vi "Scanner with R and T displays.vi"() -> ()   [LabVIEW 2012]
doc: "Application example"
uses:
  <vilib>/ptbypt/NI_PtbyPt.lvlib
panel:
  in  "EXIT W/O SAVING":bool
  out "MEASURING":i32
  out "EDIT":string
  out "SELECT":string
  out "SCAN CYCLE FINISHED":bool
  out "ADC OVERRANGE":bool
  out "UNIT":string[](array[string])
  out "RPC7":bool
  out "RPC6":bool
  out "RPC5":bool
  out "RPC4":bool
  out "RPC3":bool
  out "RPC2":bool
  out "RPC1":bool
  out "RPC0":bool
  out "T[CH]":dbl[](array[numeric]) format="%_6g"
  out "RPC":bool[](array[boolean])
  out "CURRENT TEMPERATURE":dbl caption="TEMPERATURE" format="%_5f"
  out "CH0":bool
  out "CH1":bool
  out "CH2":bool
  out "CH3":bool
  out "CH4":bool
  out "CH5":bool
  out "CH6":bool
  out "CH7":bool
  out "R[CH] OHMS":dbl[](array[numeric]) format="%_6g"
  in  "RESISTANCE":dbl format="%_5f"
  in  "SCAN SETTINGS":T1(array[cluster])=[{"SCAN ENABLED"=0, "INPUT"=0, "RANGE"=3, "AUTORANGE"=0, "EXCITATION"=0, "STAB DELAY"=0, "AVERAGE COUNT"=1}, {"SCAN ENABLED"=0, "INPUT"=0, "RANGE"=3, "AUTORANGE"=0, "EXCITATION"=0, "STAB DELAY"=0, "AVERAGE COUNT"=1}, {"SCAN ENABLED"=0, "INPUT"=0, "RANGE"=3, "AUTORANGE"=0, "EXCITATION"=0, "STAB DELAY"=0, "AVERAGE COUNT"=1}, {"SCAN ENABLED"=0, "INPUT"=0, "RANGE"=3, "AUTORANGE"=0, "EXCITATION"=0, "STAB DELAY"=0, "AVERAGE COUNT"=1}, {"SCAN ENABLED"=0, "INPUT"=0, "RANGE"=3, "AUTORANGE"=0, "EXCITATION"=0, "STAB DELAY"=0, "AVERAGE COUNT"=1}, {"SCAN ENABLED"=0, "INPUT"=0, "RANGE"=3, "AUTORANGE"=0, "EXCITATION"=0, "STAB DELAY"=0, "AVERAGE COUNT"=1}, {"SCAN ENABLED"=0, "INPUT"=0, "RANGE"=3, "AUTORANGE"=0, "EXCITATION"=0, "STAB DELAY"=0, "AVERAGE COUNT"=1}, {"SCAN ENABLED"=0, "INPUT"=0, "RANGE"=3, "AUTORANGE"=0, "EXCITATION"=0, "STAB DELAY"=0, "AVERAGE COUNT"=1}] {"SCAN ENABLED" items=["NO", "YES"]; "INPUT" items=["ZERO", "MEAS", "CAL"]; "RANGE" items=["NO RANGE", "2 Ohms", "20 Ohms", "200 Ohms", "2 kOhms", "20 kOhms", "200 kOhms", "2 MOhms"]; "AUTORANGE" items=["NO", "YES"]; "EXCITATION" items=["NO EXCITATION", "3 uV", "10uV", "30uV", "100uV", "300uV", "1mV", "3mV"]}
  in  "STOP":bool caption="PREMATURE STOPPING"
  in  "CH":i32
  in  "AVG_I":i32
  in  "START A CYCLE":bool
  in  "EXIT AND SAVE":bool
  out "SCAN FILE READ INFO":string
  # "Scanner with R and T Displays.vi"
  # "CURRENTLY MEASURING"
  # "CH"
  # "Start the VI before editing. Edits\nmade before starting are lost."
  # "R Past Calibration\nRange"
  # "Prepare the R/T calibration text files according to instructions\nPrepare information file about the calibration files using Edit RT Information File.vi\nTest the R/T conversion using Free Running Avs47b with temperature display.vi \n\nStart this VI. SCAN FILE READ INFO will be blank, if all the calibration files that are\nlisted by file avs47b_rt_file_info.cnf . \"Select Action..\" -text  should appear.\nEdit the scan settings, if needed. Enable scanning for the required channels, select suitable  \nrange and excitation for those channels. \n\n If possible, enable autoranging for each channel that will be scanned. This will prevent \nresults that include erroneous readings due to ADC overload.  After starting, autoranging\ncontinues until a valid range is found.  Then the channel is measured. If the reading\nfalls under 1800 or exceeds 19000 during averaging, range is changed downwards or\nupwards and, after a stabilisation delay, averaging starts from the beginning.\n\nStabilisation delay should be about 5 seconds for the highest excitations and about 15 \nseconds for the lowest excitation. There is a tradeoff between scanning speed and \ntime for finding good and final balance.  Required average count depends on excitation \nand the desired accuracy. \n\nWhen you are ready with editing, either save the edited (or non-edited) settings and exit, \nor start a single scan cycle. The settings will be saved after the cycle.\n\nThe scan-enabled channels are measured.  The mean values of resistances\nare output for all channels, temperatures are shown for channels that have a \ncalibration file.  Temperature unit has been specified in the scan info file.\nAfter the scan cycle, the bridge returns to its initial state. The possibly edited\nscan settings are saved."
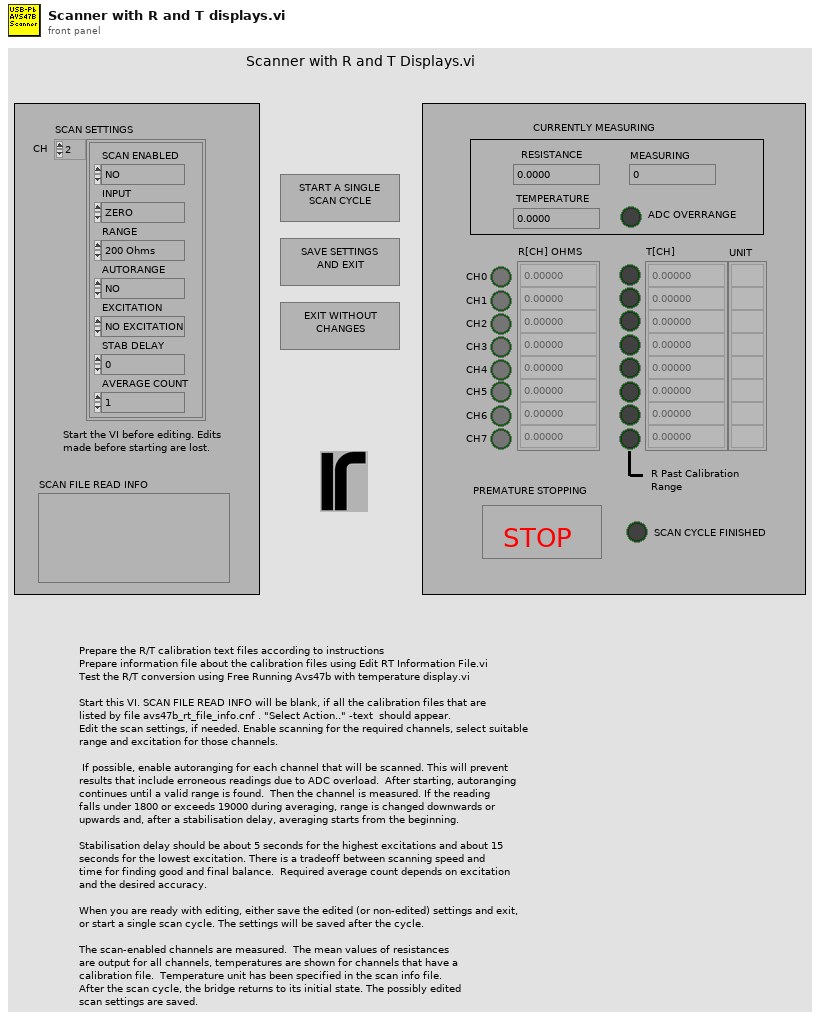
[diagram p1: front panel]
types:
  T1 = cluster{"SCAN ENABLED":u8, "INPUT":u8, "RANGE":u8, "AUTORANGE":u8, "EXCITATION":u8, "STAB DELAY":i32, "AVERAGE COUNT":i32}[]
  T2 = enum16{"NONE", "READ", "READ AND EDIT", "DEFAULTS"}
  T3 = cluster{"VISA RESOURCE":refnum<visa-resource-name>, "PICOBUS ADDRESS":u8, "DISABLE AL":u8, "REMOTE":u8, "INPUT":u8, "CHANNEL":u8, "RANGE":u8, "EXCITATION":u8, "DISPLAY":u8, "DIGITAL REFERENCE":u16, "SET POINT":dbl, "PROP GAIN":u8, "INTG":u8, "DERIV":u8, "POWER BIAS":u8, "POWER RANGE":u8, "INFO STRING":string, "HEATER RESISTANCE":dbl, "INTERVAL":u8, " SENSOR dR/dT":u8}
  T4 = cluster{"NUMBER OF POINTS":i32, "SIGN OF dT/dR":enum16{"POSITIVE", "NEGATIVE"}, "R/T FORMAT ":enum16{"R", "LOG(R)"}, "TEMPERATURE SCALE":enum16{"KELVINS", "CELSIUS"}, "FILE OK":i32}[]
  T5 = enum16{"SCAN CHECK", "CONFIGURE", "MEASURE", "CALC AVE", "READY"}
  T6 = cluster{"SCAN ENABLED":u8, "INPUT":u8, "RANGE":u8, "AUTORANGE":u8, "EXCITATION":u8, "STAB DELAY":i32, "AVERAGE COUNT":i32}
  T7 = cluster{bool, bool, bool, bool, bool, bool, bool, bool, bool, bool, bool, bool, bool, bool, bool, bool}
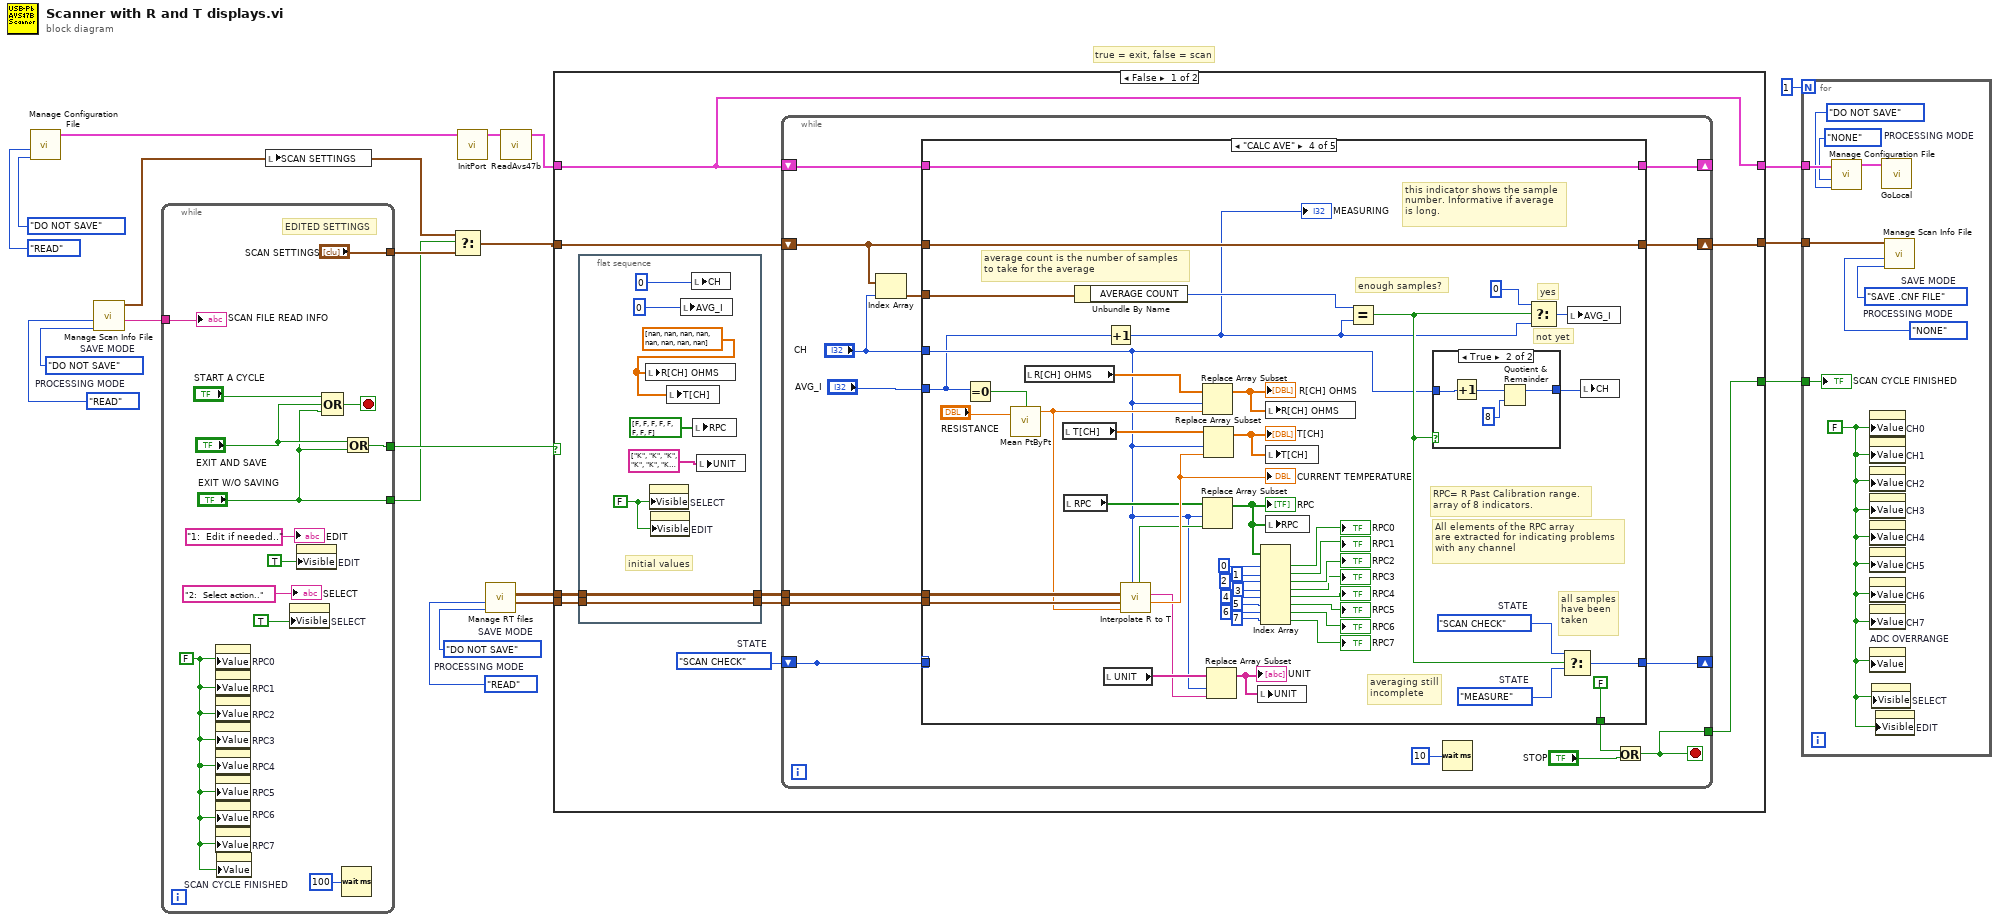
[diagram p0: block diagram]
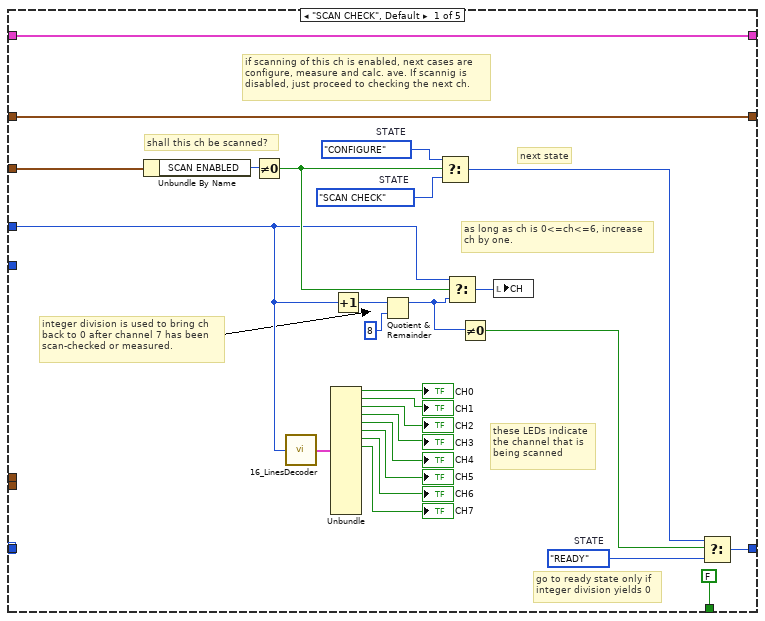
[diagram p2: hidden frame]
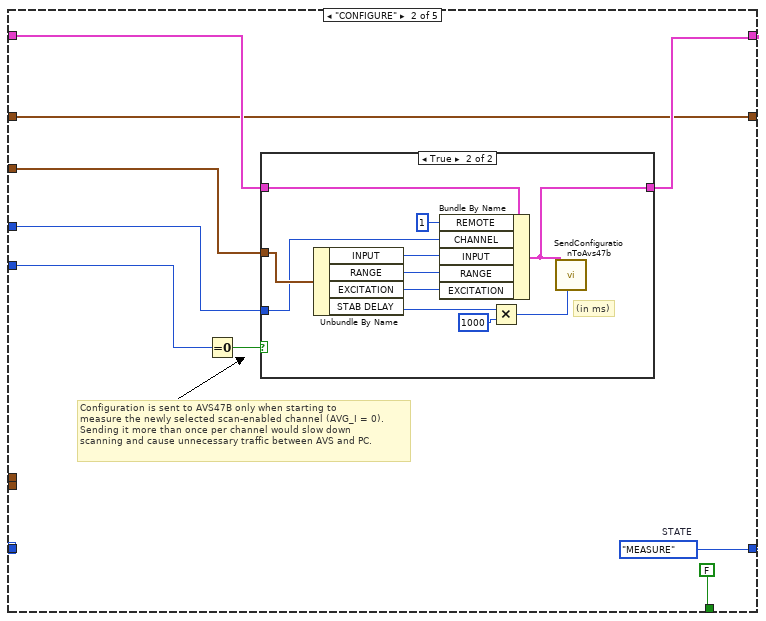
[diagram p3: hidden frame]
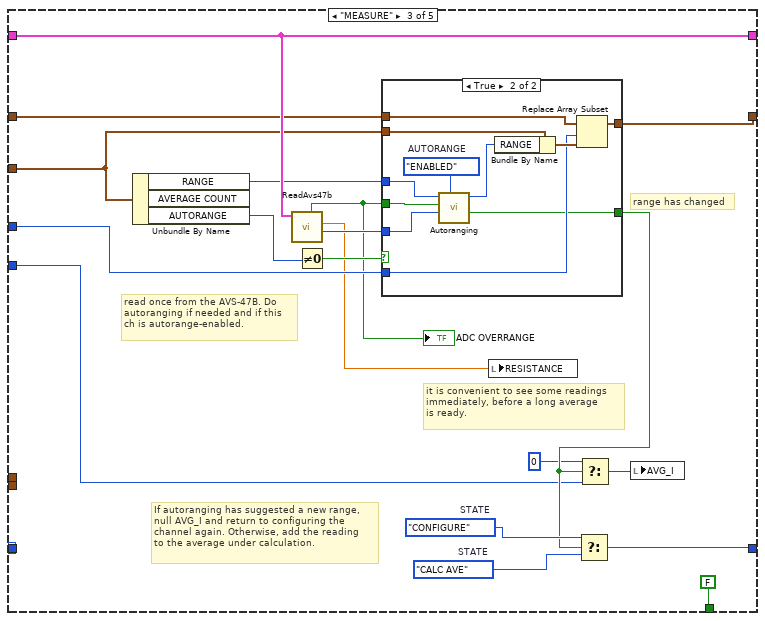
[diagram p5: hidden frame]
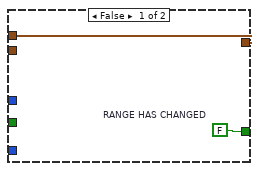
[diagram p6: hidden frame]
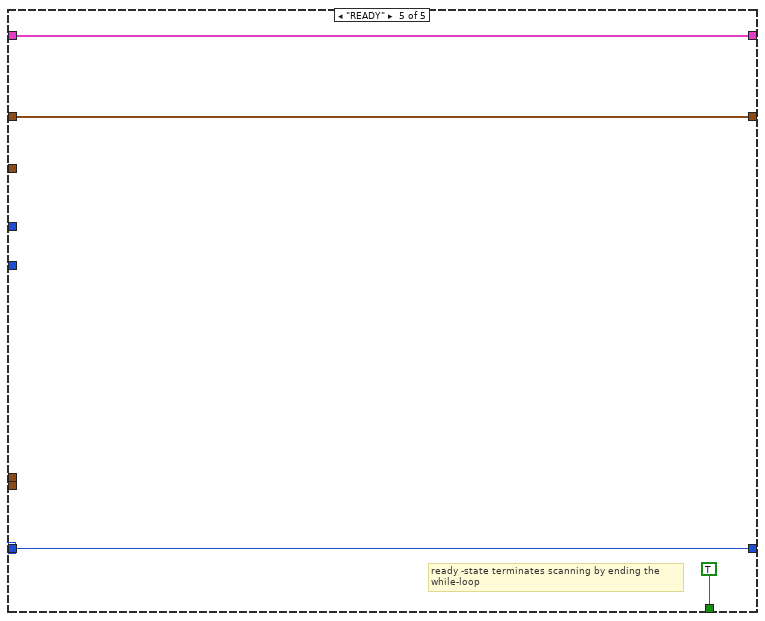
[diagram p8: hidden frame]
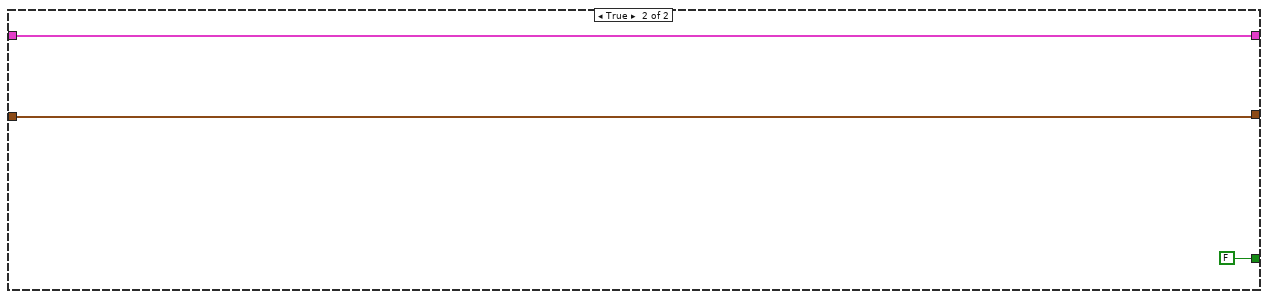
[diagram p9: hidden frame]
diagram:
  w6 = T2."READ"  # PROCESSING MODE
  w7 = enum16{"DO NOT SAVE", "SAVE .CNF FILE"}."DO NOT SAVE"  # SAVE MODE
  w10 = T2."READ"  # PROCESSING MODE
  w11 = enum16{"DO NOT SAVE", "SAVE .CNF FILE"}."DO NOT SAVE"  # SAVE MODE
  # "true = exit, false = scan"
  n1 = call "Manage Configuration File.vi"("SAVE MODE"=enum16{"DO NOT SAVE", "SAVE .CNF FILE"}."DO NOT SAVE", "PROCESSING MODE"=enum16{"NONE", "READ", "CREATE"}."READ") -> ("CONFIGURATION CLUSTER OUT"=w5:T3)  [unwired: 9 in]
  n2 = call "Manage Scan Info File.vi"("SAVE MODE"=w11, "PROCESSING MODE"=w10) -> ("SCAN FILE READ INFO"=w12:string, "SCAN INFO CLUSTER ARRAY OUT"=w3:T1)  [unwired: 7 in, 1 out]
  n3 = while {
    tunnel: [w24] -> w21
    tunnel: ["SCAN SETTINGS"] -> w4
    tunnel: w12 -> [w33]
    tunnel: ["EXIT W/O SAVING"] -> w2
    stop <- w26 stop-if-true
    w27 = FALSE ("RPC0")
    # "EDITED SETTINGS"
    n4 = property on="RPC0" class="Bool (strict)"("Value"=w27) -> ()  [unwired: 2 in, 2 out]
    n5 = property on="RPC1" class="Bool (strict)"("Value"=w27) -> ()  [unwired: 2 in, 2 out]
    n6 = property on="RPC2" class="Bool (strict)"("Value"=w27) -> ()  [unwired: 2 in, 2 out]
    n7 = property on="RPC3" class="Bool (strict)"("Value"=w27) -> ()  [unwired: 2 in, 2 out]
    n8 = property on="RPC4" class="Bool (strict)"("Value"=w27) -> ()  [unwired: 2 in, 2 out]
    n9 = property on="RPC5" class="Bool (strict)"("Value"=w27) -> ()  [unwired: 2 in, 2 out]
    n10 = property on="RPC6" class="Bool (strict)"("Value"=w27) -> ()  [unwired: 2 in, 2 out]
    n11 = property on="RPC7" class="Bool (strict)"("Value"=w27) -> ()  [unwired: 2 in, 2 out]
    n12 = property on="SCAN CYCLE FINISHED" class="Bool (strict)"("Value"=w27) -> ()  [unwired: 2 in, 2 out]
    n13 = property on="SELECT" class="Str"("Visible"=TRUE) -> ()  [unwired: 2 in, 2 out]
    n14 = property on="EDIT" class="Str"("Visible"=TRUE) -> ()  [unwired: 2 in, 2 out]
    n15 = Compound Arithmetic op=OR("START A CYCLE", "EXIT AND SAVE", "EXIT W/O SAVING") -> (w26:bool)
    n16 = Wait (ms)(milliseconds to wait=u32 100) -> ()  [unwired: 1 out]
    n17 = Or(x="EXIT AND SAVE", y="EXIT W/O SAVING") -> (x .or. y?=w24:bool)
    "SCAN FILE READ INFO" <- w33
    "EDIT" <- "1:  Edit if needed.."
    "SELECT" <- "2:  Select action.."
  }
  n18 = local write "SCAN SETTINGS"(w3) -> ()
  n19 = Select(t=w3, s=w2, f=w4) -> (s? t:f=w1:T1)
  n20 = call "InitPort.vi"("CONFIGURATION CLUSTER"=w5) -> ("UNMODIFIED CONFIGURATION CLUSTER"=w13:T3)  [unwired: 6 in, 2 out]
  n21 = call "Manage RT files.vi"("SAVE MODE"=w7, "PROCESSING MODE"=w6) -> ("FILE INFO"=w8:T4, "R/T BREAKPOINTS"=w9:cluster{dbl, dbl}[][])  [unwired: 5 in, 3 out]
  n22 = call "ReadAvs47b.vi"("CONFIGURATION CLUSTER"=w13) -> ("MODIFIED CONFIGURATION CLUSTER"=w16:T3)  [unwired: 5 in, 5 out]
  n23 = case shown="False" w21 {
    tunnel: w1 -> [w36 w203]
    tunnel: w16 -> [w42 w204]
    tunnel: [w42 w204] -> w20
    tunnel: [w35 w203] -> w19
    tunnel: w9 -> [w41 _]
    tunnel: w8 -> [w39 _]
    tunnel: [w37 FALSE] -> w17
    frame False {
      w43 = T5."SCAN CHECK"  # STATE
      n24 = flat-sequence {
        tunnel: w41 -> [w47]
        tunnel: [w47] -> w40
        tunnel: w39 -> [w46]
        tunnel: [w46] -> w38
        frame #0 {
          w44 = FALSE ("Visible")
          w49 = dbl[] [nan, nan, nan, nan, nan, nan, nan, nan]
          # "initial values"
          n25 = local write "R[CH] OHMS"(w49) -> ()
          n26 = property on="SELECT" class="Str"("Visible"=w44) -> ()  [unwired: 2 in, 2 out]
          n27 = property on="EDIT" class="Str"("Visible"=w44) -> ()  [unwired: 2 in, 2 out]
          n28 = local write "T[CH]"(w49) -> ()
          n29 = local write "AVG_I"(0 ("AVG_I")) -> ()
          n30 = local write "CH"(0 ("CH")) -> ()
          n31 = local write "RPC"(bool[] [FALSE, FALSE, FALSE, FALSE, FALSE, FALSE, FALSE, FALSE]) -> ()
          n32 = local write "UNIT"(string[] ["K", "K", "K", "K", "K", "K", "K", "K"]) -> ()
        }
      }
      n33 = while {
        shift-right: [w65] -> _
        shift-left: w43 -> [w57]
        shift-right: [w60] -> _
        shift-left: w42 -> [w61]
        shift-right: [w58] -> w35
        shift-left: w36 -> [w59]
        tunnel: w40 -> [w54]
        tunnel: w38 -> [w53]
        tunnel: [w52] -> w37
        stop <- w52 stop-if-true
        n34 = Index Array(array=w59, index="CH") -> (element=w66:T6)
        n35 = case shown="\"CALC AVE\"" w57 {
          tunnel: w61 -> [w92 w100 w132 w192 w201]
          tunnel: [w92 w97 w132 w192 w201] -> w60
          tunnel: w66 -> [w91 w101 w127 w188 _]
          tunnel: [w84 w95 w123 w184 w199] -> w65
          tunnel: "CH" -> [w67 w93 w125 w149 _]
          tunnel: "AVG_I" -> [_ w99 w116 w147 _]
          tunnel: w59 -> [w85 w96 w126 w191 w200]
          tunnel: [w85 w96 w124 w191 w200] -> w58
          tunnel: w57 -> [_ _ _ _ w199]
          tunnel: [FALSE FALSE FALSE FALSE TRUE] -> w55
          tunnel: w54 -> [_ _ _ w175 _]
          tunnel: w53 -> [_ _ _ w174 _]
          frame "SCAN CHECK", Default {
            w78 = T5."READY"  # STATE
            w79 = T5."SCAN CHECK"  # STATE
            w80 = T5."CONFIGURE"  # STATE
            # "shall this ch be scanned?"
            # "integer division is used to bring ch\nback to 0 after channel 7 has been\nscan-checked or measured."
            # "go to ready state only if\ninteger division yields 0"
            # "next state"
            # "as long as ch is 0<=ch<=6, increase\nch by one."
            # "if scanning of this ch is enabled, next cases are\nconfigure, measure and calc. ave. If scannig is \ndisabled, just proceed to checking the next ch."
            # "these LEDs indicate\nthe channel that is\nbeing scanned"
            n36 = Unbundle By Name(w91) -> ("SCAN ENABLED"=w90:u8)
            n37 = Not Equal To 0?(x=w90) -> (x != 0?=w87:bool)
            n38 = call "16_LinesDecoder.vi"("Integer 0..15  (0)"=w67) -> ("decoded drives"=w76:T7)  [unwired: 4 in]
            n39 = Unbundle(w76) -> (→"CH0":bool, →"CH1":bool, →"CH2":bool, →"CH3":bool, →"CH4":bool, →"CH5":bool, →"CH6":bool, →"CH7":bool)  [unwired: 8 out]
            n40 = Increment(x=w67) -> (x+1=w89:i32)
            n41 = Quotient & Remainder(x=w89, y=8) -> (x-y*floor(x/y)=w82:i32)  [unwired: 1 out]
            n42 = Select(t=w80, s=w87, f=w79) -> (s? t:f=w83:T5)
            n43 = Select(t=w67, s=w87, f=w82) -> (s? t:f=w86:i32)
            n44 = Not Equal To 0?(x=w82) -> (x != 0?=w81:bool)
            n45 = local write "CH"(w86) -> ()
            n46 = Select(t=w83, s=w81, f=w78) -> (s? t:f=w84:T5)
          }
          frame "CONFIGURE" {
            w95 = T5."MEASURE"  # STATE
            # "Configuration is sent to AVS47B only when starting to \nmeasure the newly selected scan-enabled channel (AVG_I = 0).\nSending it more than once per channel would slow down \nscanning and cause unnecessary traffic between AVS and PC."
            n47 = Equal To 0?(x=w99) -> (x = 0?=w98:bool)
            n48 = case shown="True" w98 {
              tunnel: w101 -> [_ w113]
              tunnel: w93 -> [_ w109]
              tunnel: w100 -> [w102 w105]
              tunnel: [w102 w104] -> w97
              frame False {
              }
              frame True {
                # "(in ms)"
                n49 = Unbundle By Name(w113) -> ("INPUT"=w112:u8, "RANGE"=w111:u8, "EXCITATION"=w110:u8, "STAB DELAY"=w108:i32)
                n50 = Bundle By Name(cluster=w105, "REMOTE"=u8 1, "CHANNEL"=w109, "INPUT"=w112, "RANGE"=w111, "EXCITATION"=w110) -> (w104:T3)
                n51 = Multiply(x=w108, y=1000) -> (x*y=w106:i32)
                n52 = call "SendConfigurationToAvs47b.vi"("STABILISATION DELAY (ms)"=w106, "CONFIGURATION CLUSTER"=w104) -> ()  [unwired: 6 in, 4 out]
              }
            }
          }
          frame "MEASURE" {
            w120 = T5."CALC AVE"  # STATE
            w121 = T5."CONFIGURE"  # STATE
            # "If autoranging has suggested a new range,\nnull AVG_I and return to configuring the \nchannel again. Otherwise, add the reading\nto the average under calculation."
            # "it is convenient to see some readings \nimmediately, before a long average\nis ready."
            # "read once from the AVS-47B. Do\nautoranging if needed and if this\nch is autorange-enabled."
            # "range has changed"
            n53 = Unbundle By Name(w127) -> ("RANGE"=w128:u8, "AUTORANGE"=w131:u8)  [unwired: 1 out]
            n54 = call "ReadAvs47b.vi"("CONFIGURATION CLUSTER"=w132) -> ("ADC"=w129:i32, "RESISTANCE (OHMS)"=w122:sgl, "ADC OVERRANGE"=w118:bool)  [unwired: 5 in, 3 out]
            "ADC OVERRANGE" <- w118
            n55 = Not Equal To 0?(x=w131) -> (x != 0?=w130:bool)
            n56 = case shown="True" w130 {
              tunnel: w129 -> [_ w145]
              tunnel: w128 -> [_ w144]
              tunnel: w118 -> [_ w143]
              tunnel: w127 -> [_ w142]
              tunnel: w126 -> [w134 w140]
              tunnel: w125 -> [_ w138]
              tunnel: [w134 w137] -> w124
              tunnel: [w133 w136] -> w117
              frame False {
                w133 = FALSE  # RANGE HAS CHANGED
              }
              frame True {
                w135 = enum16{"DISABLED", "ENABLED"}."ENABLED"  # AUTORANGE
                n57 = call "Autoranging.vi"("AUTORANGE"=w135, "ADC"=w145, "OVR"=w143, "RANGE"=w144) -> ("RANGE HAS CHANGED"=w136:bool, "NEW RANGE"=w141:i32)  [unwired: 4 in, 2 out]
                n58 = Bundle By Name(cluster=w142, "RANGE"=w141) -> (w139:T6)
                n59 = Replace Array Subset(array=w140, new element=w139, index=w138) -> (w137:T1)
              }
            }
            n60 = local write "RESISTANCE"(w122) -> ()
            n61 = Select(t=w121, s=w117, f=w120) -> (s? t:f=w123:T5)
            n62 = Select(t=0, s=w117, f=w116) -> (s? t:f=w114:i32)
            n63 = local write "AVG_I"(w114) -> ()
          }
          frame "CALC AVE" {
            w180 = T5."MEASURE"  # STATE
            w181 = T5."SCAN CHECK"  # STATE
            # "all samples\nhave been\ntaken"
            # "averaging still\nincomplete"
            # "All elements of the RPC array\nare extracted for indicating problems\nwith any channel"
            # "RPC= R Past Calibration range.\narray of 8 indicators."
            # "not yet"
            # "yes"
            # "enough samples?"
            # "average count is the number of samples\nto take for the average"
            # "this indicator shows the sample\nnumber. Informative if average\nis long."
            n64 = Equal To 0?(x=w147) -> (x = 0?=w189:bool)
            n65 = call <vilib>:"Mean PtByPt.vi"("x"="RESISTANCE", "initialize"=w189) -> ("mean"=w173:dbl)  [unwired: 2 in, 1 out]
            n66 = local read "R[CH] OHMS"() -> (w178:dbl[])
            n67 = local read "T[CH]"() -> (w176:dbl[])
            n68 = local read "RPC"() -> (w170:bool[])
            n69 = Unbundle By Name(w188) -> ("AVERAGE COUNT"=w187:i32)
            n70 = local read "UNIT"() -> (w151:string[])
            n71 = Increment(x=w147) -> (x+1=w146:i32)
            "MEASURING" <- w146
            n72 = call "Interpolate R to T.vi"("CHANNEL"=w149, "RESISTANCE (OHMS)"=w173, "FILE INFO"=w174, "R/T POINTS"=w175) -> ("TEMPERATURE"=w171:dbl, "TEMPERATURE UNIT"=w150:string, "R PAST CALIBRATION RANGE"=w169:bool)  [unwired: 4 in, 1 out]
            "CURRENT TEMPERATURE" <- w171
            n73 = Replace Array Subset(array=w178, new element=w173, index=w149) -> (w177:dbl[])
            "R[CH] OHMS" <- w177
            n74 = Replace Array Subset(array=w170, new element=w169, index=w149) -> (w168:bool[])
            "RPC" <- w168
            n75 = Replace Array Subset(array=w176, new element=w171, index=w149) -> (w172:dbl[])
            "T[CH]" <- w172
            n76 = Replace Array Subset(array=w151, new element=w150, index=w149) -> (w148:string[])
            "UNIT" <- w148
            n77 = local write "UNIT"(w148) -> ()
            n78 = Index Array(array=w168, index #1=0 ("index"), index #2=1 ("index"), index #3=2 ("index"), index #4=3 ("index"), index #5=4 ("index"), index #6=5 ("index"), index #7=6 ("index"), index #8=7 ("index")) -> (element #1=→"RPC0":bool, element #2=→"RPC1":bool, element #3=→"RPC2":bool, element #4=→"RPC3":bool, element #5=→"RPC4":bool, element #6=→"RPC5":bool, element #7=→"RPC6":bool, element #8=→"RPC7":bool)
            n79 = local write "R[CH] OHMS"(w177) -> ()
            n80 = local write "T[CH]"(w172) -> ()
            n81 = local write "RPC"(w168) -> ()
            n82 = Equal?(x=w187, y=w146) -> (x = y?=w183:bool)
            n83 = case shown="True" w183 {
              tunnel: w149 -> [w193 w195]
              tunnel: [w193 w194] -> w182
              frame False {
              }
              frame True {
                n84 = Increment(x=w195) -> (x+1=w197:i32)
                n85 = Quotient & Remainder(x=w197, y=8) -> (x-y*floor(x/y)=w194:i32)  [unwired: 1 out]
              }
            }
            n86 = Select(t=0, s=w183, f=w146) -> (s? t:f=w185:i32)
            n87 = Select(t=w181, s=w183, f=w180) -> (s? t:f=w184:T5)
            n88 = local write "AVG_I"(w185) -> ()
            n89 = local write "CH"(w182) -> ()
          }
          frame "READY" {
            # "ready -state terminates scanning by ending the \nwhile-loop"
          }
        }
        n90 = Wait (ms)(milliseconds to wait=u32 10) -> ()  [unwired: 1 out]
        n91 = Or(x=w55, y="STOP") -> (x .or. y?=w52:bool)
      }
    }
    frame True {
    }
  }
  n92 = for {
    N: 1 -> [_]
    tunnel: w20 -> [w210]
    tunnel: w19 -> [w207]
    tunnel: w17 -> [w213]
    w205 = T2."NONE"  # PROCESSING MODE
    w206 = enum16{"DO NOT SAVE", "SAVE .CNF FILE"}."SAVE .CNF FILE"  # SAVE MODE
    w209 = enum16{"NONE", "READ", "CREATE"}."NONE"  # PROCESSING MODE
    w212 = FALSE ("RPC0")
    n93 = call "Manage Configuration File.vi"("SAVE MODE"=enum16{"DO NOT SAVE", "SAVE .CNF FILE"}."DO NOT SAVE", "PROCESSING MODE"=w209, "CONFIGURATION CLUSTER"=w210) -> ("CONFIGURATION CLUSTER OUT"=w211:T3)  [unwired: 8 in]
    n94 = property on="CH0" class="Bool (strict)"("Value"=w212) -> ()  [unwired: 2 in, 2 out]
    n95 = property on="CH1" class="Bool (strict)"("Value"=w212) -> ()  [unwired: 2 in, 2 out]
    n96 = property on="CH2" class="Bool (strict)"("Value"=w212) -> ()  [unwired: 2 in, 2 out]
    n97 = property on="CH3" class="Bool (strict)"("Value"=w212) -> ()  [unwired: 2 in, 2 out]
    n98 = property on="CH4" class="Bool (strict)"("Value"=w212) -> ()  [unwired: 2 in, 2 out]
    n99 = property on="CH5" class="Bool (strict)"("Value"=w212) -> ()  [unwired: 2 in, 2 out]
    n100 = property on="CH6" class="Bool (strict)"("Value"=w212) -> ()  [unwired: 2 in, 2 out]
    n101 = property on="CH7" class="Bool (strict)"("Value"=w212) -> ()  [unwired: 2 in, 2 out]
    n102 = property on="ADC OVERRANGE" class="Bool (strict)"("Value"=w212) -> ()  [unwired: 2 in, 2 out]
    n103 = property on="SELECT" class="Str"("Visible"=w212) -> ()  [unwired: 2 in, 2 out]
    n104 = property on="EDIT" class="Str"("Visible"=w212) -> ()  [unwired: 2 in, 2 out]
    n105 = call "GoLocal.vi"("CONFIGURATION CLUSTER"=w211) -> ()  [unwired: 10 in, 1 out]
    n106 = call "Manage Scan Info File.vi"("SAVE MODE"=w206, "PROCESSING MODE"=w205, "SCAN INFO CLUSTER ARRAY IN"=w207) -> ()  [unwired: 6 in, 3 out]
    "SCAN CYCLE FINISHED" <- w213
  }
